vi "GenerateNavigationPages.vi"(2 "Root Directory":path, 3 "VI Documentation Pages":path[](array[path]), 4 "Project name":string="<Project Name>") -> ()   [LabVIEW 2018, in "ArgosLib.lvlib"]
uses:
  ArgosLib.lvlib
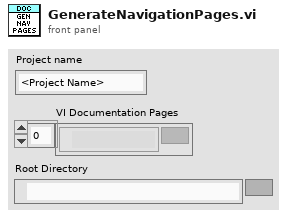
[diagram p1: front panel]
types:
  T1 = enum16{"open", "replace", "create", "open or create", "replace or create", "replace or create with confirmation"}
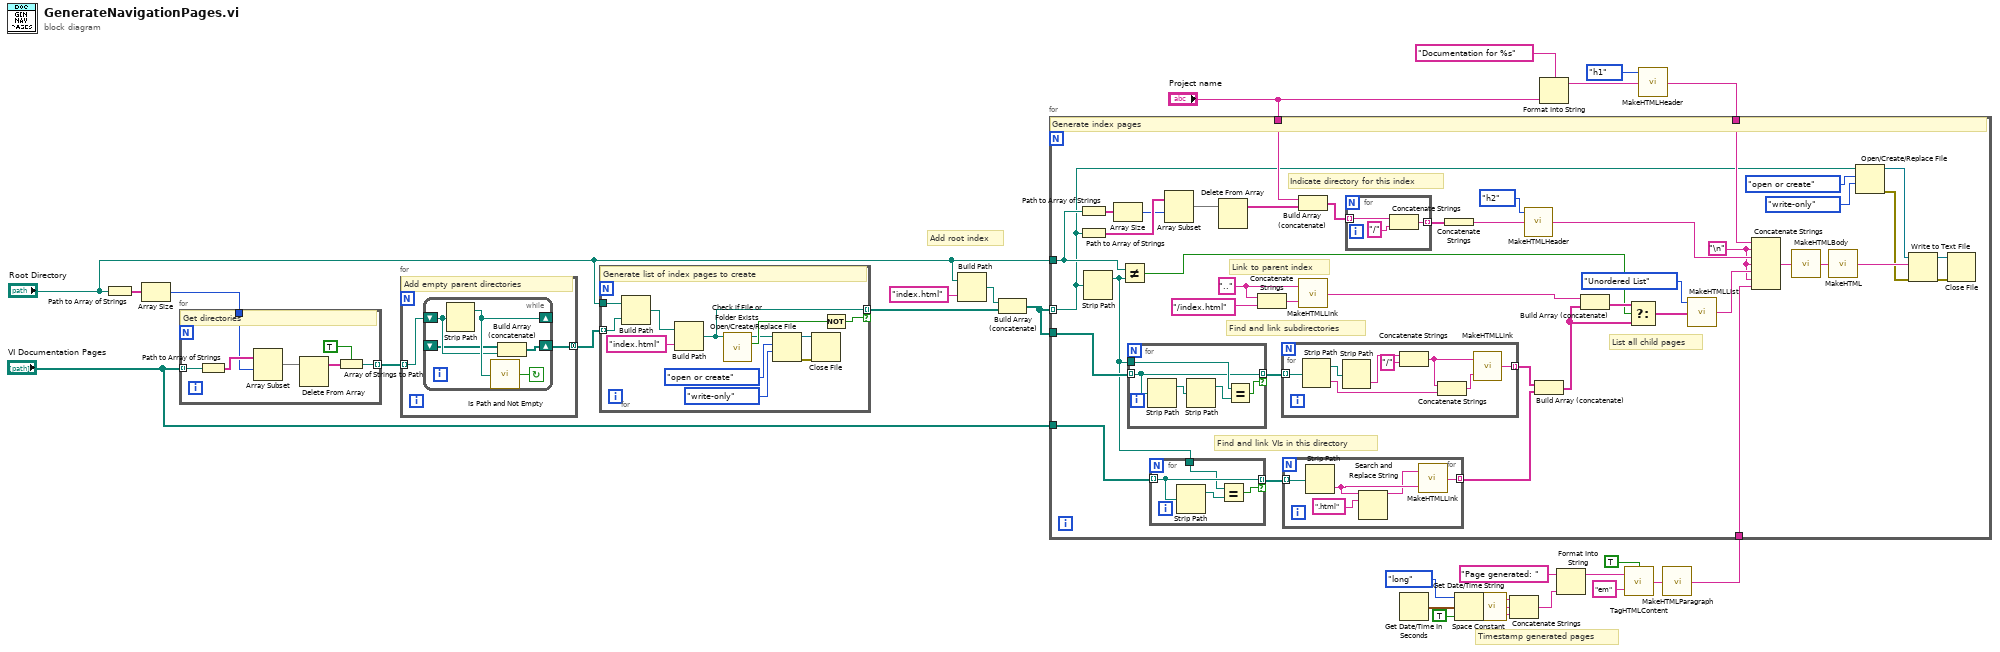
[diagram p0: block diagram]
diagram:
  # "Timestamp generated pages"
  # "Add root index"
  n1 = Path to Array of Strings(0:"Root Directory") -> (2:w28:string[])  [unwired: 1 out]
  n2 = Array Size(array=w28) -> (size(s)=w27:i32)
  n3 = for {
    tunnel: "VI Documentation Pages" -> [w35] mode=indexing
    tunnel: w27 -> [w33]
    tunnel: [w30] -> w2 mode=indexing
    # "Get directories"
    n4 = Path to Array of Strings(0:w35) -> (2:w34:string[])  [unwired: 1 out]
    n5 = Array Subset(array=w34, index=w33) -> (w32:string[])  [unwired: 1 in]
    n6 = Delete From Array(array=w32) -> (array with subset deleted=w31:string[])  [unwired: 2 in, 1 out]
    n7 = Array of Strings to Path(0:w31, 1:TRUE ("relative")) -> (2:w30:path)
  }
  n8 = for {
    tunnel: w2 -> [w37] mode=indexing
    tunnel: [w36] -> w1 mode=concatenating
    # "Add empty parent directories"
    n9 = while {
      shift-right: [w41] -> _
      shift-left: w37 -> [w40]
      shift-right: [w39] -> w36
      shift-left: _ -> [w38]
      stop <- w42 continue-if-true
      n10 = Strip Path(path=w40) -> (stripped path=w41:path)  [unwired: 1 out]
      n11 = call <vilib>:"Is Path and Not Empty.vi"("path"=w41) -> ("Is Path and Not Empty?"=w42:bool)  [unwired: 4 in]
      n12 = Build Array (concatenate)(w38, w40) -> (w39:path[])
    }
  }
  n13 = for {
    tunnel: w1 -> [w54] mode=indexing
    tunnel: "Root Directory" -> [w53]
    tunnel: [w50] -> w7 mode=indexing if=w49
    # "Generate list of index pages to create"
    n14 = Build Path(base path=w53, name or relative path=w54) -> (appended path=w52:path)
    n15 = Build Path(base path=w52, name or relative path="index.html") -> (appended path=w50:path)
    n16 = call <vilib>:"Check if File or Folder Exists.vi"("path"=w50) -> ("file or folder exists?"=w48:bool, "dup path"=w47:path)  [unwired: 8 in, 1 out]
    n17 = Open/Create/Replace File(file path (use dialog)=w47, operation (0:open)=T1."open or create", access (0:read/write)=enum16{"read/write", "read-only", "write-only"}."write-only") -> (refnum out=w43:refnum<file>, error out=w44:errorcluster)  [unwired: 3 in, 1 out]
    n18 = Close File(refnum=w43, error in=w44) -> ()  [unwired: 2 out]
    n19 = Not(x=w48) -> (.not. x?=w49:bool)
  }
  n20 = Build Path(base path="Root Directory", name or relative path="index.html") -> (appended path=w5:path)
  n21 = Build Array (concatenate)(w5, w7) -> (w6:path[])
  n22 = Get Date/Time In Seconds() -> (seconds since 1Jan1904=w22:timestamp)
  n23 = Get Date/Time String(date format (0)=enum16{"short", "long", "abbreviated"}."long", seconds (now)=w22, want seconds? (F)=TRUE) -> (date string=w21:string, time string=w20:string)
  n24 = call <vilib>:"Space Constant.vi"() -> ("String"=w19:string)
  n25 = Concatenate Strings(w21, w19, w20) -> (w17:string)
  n26 = Format Into String(format string="Documentation for %s", "Project name") -> (resulting string=w24:string)  [unwired: 2 in, 1 out]
  n27 = Format Into String(initial string="Page generated: ", w17) -> (resulting string=w14:string)  [unwired: 2 in, 1 out]
  n28 = call "TagHTMLContent.vi"("Escape Contents"=TRUE, "Tag"="em", "Element Contents"=w14) -> ("Tagged Contents"=w12:string)
  n29 = call "MakeHTMLHeader.vi"("Header Content"=w24, "Header Type"=enum16{"h1", "h2", "h3", "h4", "h5", "h6"}."h1") -> ("Header Element"=w11:string)  [unwired: 3 in]
  n30 = call "MakeHTMLParagraph.vi"("Paragraph Content"=w12) -> ("Paragraph Element"=w10:string)  [unwired: 4 in]
  n31 = for {
    tunnel: w11 -> [w68]
    tunnel: w10 -> [w79]
    tunnel: w6 -> [w64] mode=indexing
    tunnel: w6 -> [w95]
    tunnel: "VI Documentation Pages" -> [w96]
    tunnel: "Root Directory" -> [w78]
    tunnel: "Project name" -> [w74]
    w67 = "\n"
    w87 = ".." ("string")
    # "Indicate directory for this index"
    # "Link to parent index"
    # "Find and link subdirectories"
    # "Find and link VIs in this directory"
    # "List all child pages"
    # "Generate index pages"
    n32 = Path to Array of Strings(0:w78) -> (2:w77:string[])  [unwired: 1 out]
    n33 = Path to Array of Strings(0:w64) -> (2:w76:string[])  [unwired: 1 out]
    n34 = Strip Path(path=w64) -> (stripped path=w94:path)  [unwired: 1 out]
    n35 = Array Size(array=w77) -> (size(s)=w75:i32)
    n36 = Not Equal?(x=w78, y=w94) -> (x != y?=w83:bool)
    n37 = for {
      tunnel: w95 -> [w114] mode=indexing
      tunnel: w94 -> [w115]
      tunnel: [w114] -> w93 mode=indexing if=w113
      n38 = Strip Path(path=w114) -> (stripped path=w117:path)  [unwired: 1 out]
      n39 = Strip Path(path=w117) -> (stripped path=w116:path)  [unwired: 1 out]
      n40 = Equal?(x=w115, y=w116) -> (x = y?=w113:bool)
    }
    n41 = for {
      tunnel: w96 -> [w121] mode=indexing
      tunnel: w94 -> [w119]
      tunnel: [w121] -> w92 mode=indexing if=w118
      n42 = Strip Path(path=w121) -> (stripped path=w120:path)  [unwired: 1 out]
      n43 = Equal?(x=w119, y=w120) -> (x = y?=w118:bool)
    }
    n44 = Array Subset(array=w76, index=w75) -> (w56:string[])  [unwired: 1 in]
    n45 = Delete From Array(array=w56) -> (array with subset deleted=w55:string[])  [unwired: 2 in, 1 out]
    n46 = Concatenate Strings(w87, "/index.html" ("string")) -> (w86:string)
    n47 = for {
      tunnel: w93 -> [w112] mode=indexing
      tunnel: [w105] -> w91 mode=indexing
      n48 = Strip Path(path=w112) -> (stripped path=w111:path, name=w108:string)
      n49 = Strip Path(path=w111) -> (name=w110:string)  [unwired: 1 out]
      n50 = Concatenate Strings(w110, "/" ("string")) -> (w106:string)
      n51 = Concatenate Strings(w106, w108) -> (w107:string)
      n52 = call "MakeHTMLLink.vi"("Link Target"=w107, "Link Text"=w106) -> ("HTML Link"=w105:string)
    }
    n53 = for {
      tunnel: w92 -> [w104] mode=indexing
      tunnel: [w100] -> w90 mode=indexing
      n54 = Strip Path(path=w104) -> (name=w102:string)  [unwired: 1 out]
      n55 = Search and Replace String(input string=w102, search string=".html") -> (result string=w101:string)  [unwired: 6 in, 3 out]
      n56 = call "MakeHTMLLink.vi"("Link Target"=w102, "Link Text"=w101) -> ("HTML Link"=w100:string)
    }
    n57 = Build Array (concatenate)(w74, w55) -> (w73:string[])
    n58 = call "MakeHTMLLink.vi"("Link Target"=w86, "Link Text"=w87) -> ("HTML Link"=w85:string)
    n59 = for {
      tunnel: w73 -> [w99] mode=indexing
      tunnel: [w97] -> w72 mode=indexing
      n60 = Concatenate Strings(w99, "/" ("string")) -> (w97:string)
    }
    n61 = Concatenate Strings(w72) -> (w70:string)
    n62 = call "MakeHTMLHeader.vi"("Header Content"=w70, "Header Type"=enum16{"h1", "h2", "h3", "h4", "h5", "h6"}."h2") -> ("Header Element"=w69:string)  [unwired: 3 in]
    n63 = Build Array (concatenate)(w91, w90) -> (w82:string[])
    n64 = Build Array (concatenate)(w85, w82) -> (w84:string[])
    n65 = Select(t=w84, s=w83, f=w82) -> (s? t:f=w81:string[])
    n66 = call "MakeHTMLList.vi"("List Elements"=w81, "List Type"=enum16{"Ordered List", "Unordered List"}."Unordered List") -> ("List"=w80:string)  [unwired: 3 in]
    n67 = Concatenate Strings(w68, w67, w69, w67, w80, w67, w79) -> (w65:string)
    n68 = call "MakeHTMLBody.vi"("Body Content"=w65) -> ("Body Element"=w66:string)  [unwired: 4 in]
    n69 = call "MakeHTML.vi"("HTML Content"=w66) -> ("HTML Element"=w61:string)  [unwired: 4 in]
    n70 = Open/Create/Replace File(file path (use dialog)=w64, operation (0:open)=T1."open or create", access (0:read/write)=enum16{"read/write", "read-only", "write-only"}."write-only") -> (refnum out=w60:refnum<file>, error out=w57:errorcluster)  [unwired: 3 in, 1 out]
    n71 = Write to Text File(file (use dialog)=w60, text=w61, error in=w57) -> (refnum out=w58:refnum<file>, error out=w59:errorcluster)  [unwired: 1 in, 1 out]
    n72 = Close File(refnum=w58, error in=w59) -> ()  [unwired: 2 out]
  }
